vi "全局变量.vi"() -> ()   [LabVIEW 2011]
panel:
  out "Counter_Edge":i32
  out "Counter_Overflow":i32
  out "Counter_Width":i32
  in  "Complete_Flag":bool
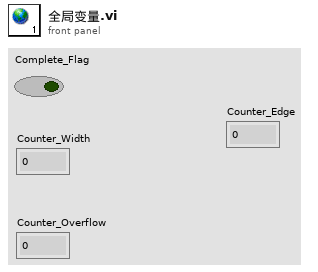
[diagram p1: front panel]
diagram:
